vi "Analog_IO_Example.vi"() -> ()   [LabVIEW 2020]
uses:
  <vilib>/Galil/resources/gclib/gclib.lvlib
panel:
  in  "File Path":path=path "Select a easy to find location for storing your .txt file"
  in  "IP Address":string="192.168.1.77"
  out "Analog Input 1":string=" 2.5851\r\n:"
  in  "stop":bool
  out "error out":errorcluster
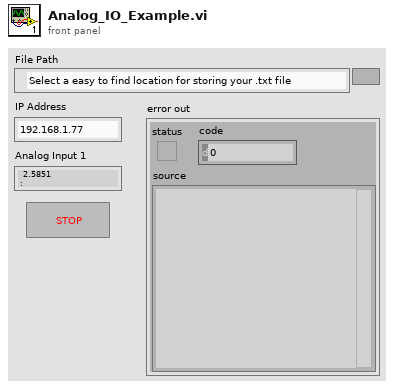
[diagram p1: front panel]
types:
  T1 = enum16{"open", "replace", "create", "open or create", "replace or create", "replace or create with confirmation"}
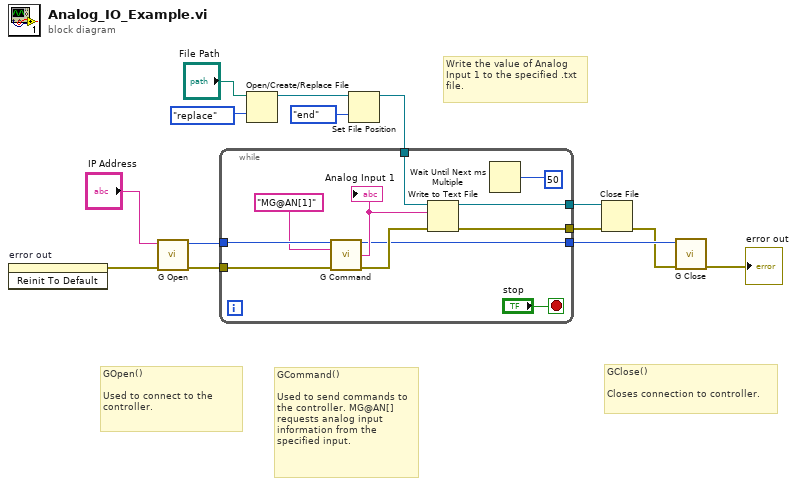
[diagram p0: block diagram]
diagram:
  # "Write the value of Analog Input 1 to the specified .txt file."
  # "GCommand()\n\nUsed to send commands to the controller. MG@AN[] requests analog input information from the specified input."
  # "GClose()\n\nCloses connection to controller."
  # "GOpen()\n\nUsed to connect to the controller."
  n1 = invoke on="error out" class="Clust (strict)" method="Reinit To Default"() -> (error out=w3:errorcluster)  [unwired: 3 in, 2 out]
  n2 = call <vilib>:"G Open.vi"("error in (no error)"=w3, "address"="IP Address") -> ("error out"=w2:errorcluster, "g out"=w1:u64)  [unwired: 7 in]
  n3 = Open/Create/Replace File(file path (use dialog)="File Path", operation (0:open)=T1."replace") -> (refnum out=w10:refnum<file>)  [unwired: 4 in, 2 out]
  n4 = Set File Position(refnum=w10, from (0:start)=enum16{"start", "end", "current"}."end") -> (refnum out=w5:refnum<file>)  [unwired: 2 in, 1 out]
  n5 = while {
    tunnel: [w15] -> w13
    tunnel: w1 -> [w20]
    tunnel: w2 -> [w18]
    tunnel: [w23] -> w8
    tunnel: [w22] -> w7
    tunnel: w5 -> [w21]
    stop <- "stop" stop-if-true
    n6 = call <vilib>:"G Command.vi"("g"=w20, "command"="MG@AN[1]" ("buffer"), "error in (no error)"=w18) -> ("g out"=w15:u64, "buffer out"=w16:string, "error out"=w17:errorcluster)  [unwired: 10 in]
    "Analog Input 1" <- w16
    n7 = Write to Text File(file (use dialog)=w21, text=w16, error in=w17) -> (refnum out=w23:refnum<file>, error out=w22:errorcluster)  [unwired: 1 in, 1 out]
    n8 = Wait Until Next ms Multiple(millisecond multiple=u32 50) -> ()  [unwired: 1 out]
  }
  n9 = Close File(refnum=w8, error in=w7) -> (error out=w6:errorcluster)  [unwired: 1 out]
  n10 = call <vilib>:"G Close.vi"("error in (no error)"=w6, "g"=w13) -> ("error out"=→"error out":errorcluster)  [unwired: 9 in]
